vi "Force_read_write_priveliges.vi"() -> ()   [LabVIEW 2013]
uses:
  <vilib>/addons/database/_DB Variant To Data/Database Variant To Data.xnode
panel:
  in  "Min timestamp":i64=1438964522810
  out "Query in Standard Format":string
  out "error out":errorcluster
  in  "error in (no error)":errorcluster
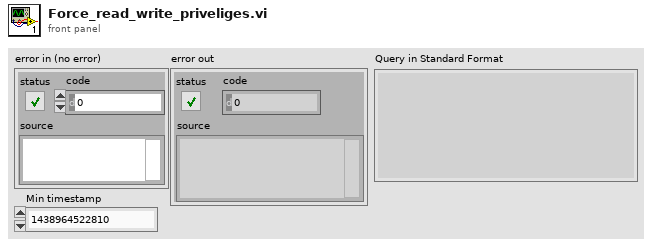
[diagram p1: front panel]
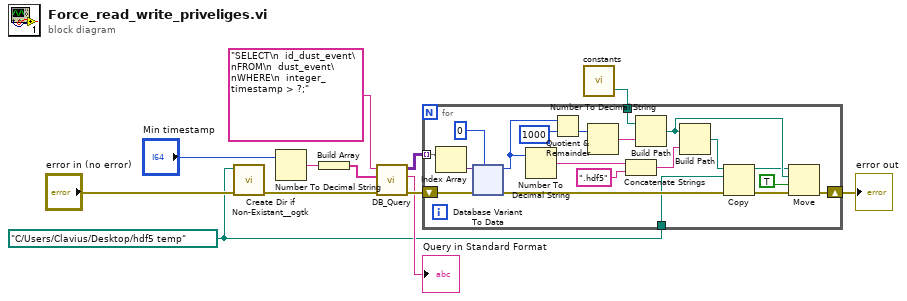
[diagram p0: block diagram]
diagram:
  w1 = path "C:/Users/Clavius/Desktop/hdf5 temp" ("target path (use dialog)")
  n1 = call <userlib>:"Create Dir if Non-Existant__ogtk.vi"("error in (no error)"="error in (no error)", "Directory Path"=w1) -> ("error out"=w2:errorcluster)  [unwired: 7 in, 2 out]
  n2 = Number To Decimal String(number="Min timestamp") -> (decimal integer string=w11:string)  [unwired: 1 in]
  n3 = Build Array(w11) -> (w10:string[])
  n4 = call <userlib>:"DB_Query.vi"("error in (no error)"=w2, "Parameters"=w10, "Parameterized Query"="SELECT\n  id_dust_event\nFROM\n  dust_event\nWHERE\n  integer_timestamp > ?;") -> ("error out"=w8:errorcluster, "Query in Standard Format"=→"Query in Standard Format":string, "Results"=w7:variant[][])  [unwired: 6 in]
  n5 = call <userlib>:"constants.vi"() -> ("Processed HDF5 filepath"=w4:path)  [unwired: 3 out]
  n6 = for {
    shift-right: [w17] -> w5
    shift-left: w8 -> [w32]
    tunnel: w7 -> [w30] mode=indexing
    tunnel: w4 -> [w25]
    tunnel: w1 -> [w13]
    n7 = Index Array(array=w30) -> (element=w31:variant)  [unwired: 1 in]
    n8 = xnode "Database Variant To Data"("database variant"=w31, "error in (no error)"=w32, "type"=i64 0) -> ("data"=w26:i64, "error out"=w20:errorcluster)
    n9 = Number To Decimal String(number=w26) -> (decimal integer string=w23:string)  [unwired: 1 in]
    n10 = Quotient & Remainder(x=w26, y=1000) -> (floor(x/y)=w27:i64)  [unwired: 1 out]
    n11 = Number To Decimal String(number=w27) -> (decimal integer string=w24:string)  [unwired: 1 in]
    n12 = Concatenate Strings(w23, ".hdf5" ("string")) -> (w22:string)
    n13 = Build Path(base path=w25, name or relative path=w24) -> (appended path=w16:path)
    n14 = Build Path(base path=w16, name or relative path=w22) -> (appended path=w19:path)
    n15 = Copy(8:w20, 10:w13, 11:w19) -> (0:w18:errorcluster, 3:w15:path)  [unwired: 2 in, 1 out]
    n16 = Move(source path=w15, error in=w18, 9:TRUE ("overwrite (F)"), 10:w16) -> (error out=w17:errorcluster)  [unwired: 1 in, 2 out]
  }
  "error out" <- w5
